vi "Send Set PID Gains Msg.vi"(8 "error in (no error)":errorcluster, 10 "PID gains":T1, 11 "Message Queue in":refnum<queue>) -> (0 "error out":errorcluster, 3 "Message Queue out":refnum<queue>)   [LabVIEW 2024, in "PID Loop.lvlib" / "Set PID Gains Msg.lvclass"]
uses:
  Set PID Gains Msg.lvclass
  Set PID Gains Msg.lvclass/Set PID Gains Msg.ctl
  C:/Users/uspoaotto/OneDrive - Oregon Tool/Desktop/working copies/zeroTimeoutMessageHandler/samples/PID Controller/PID Loop/PID Loop/Set PID Gains Msg/Set PID Gains Msg.lvclass
  C:/Users/uspoaotto/OneDrive - Oregon Tool/Desktop/working copies/zeroTimeoutMessageHandler/src/Zero Timeout Message Handler/~Message/~Message.lvclass
  src/Zero Timeout Message Handler/~Message/~Message.lvclass
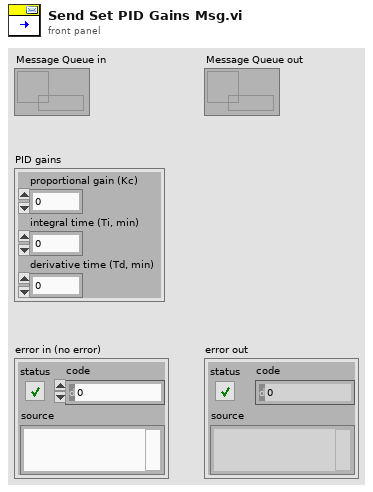
[diagram p1: front panel]
types:
  T1 = cluster{"proportional gain (Kc)":dbl, "integral time (Ti, min)":dbl, "derivative time (Td, min)":dbl}
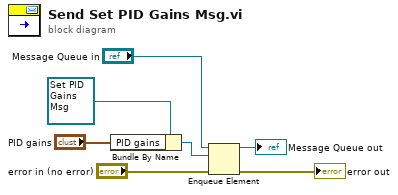
[diagram p0: block diagram]
diagram:
  n1 = Bundle By Name(cluster=refnum<class "Set PID Gains Msg.lvclass"> refnum ("PID Loop.lvlib:Set PID Gains Msg.lvclass"), "PID gains"="PID gains") -> (w1:refnum<class "Set PID Gains Msg.lvclass">)
  n2 = Enqueue Element(queue="Message Queue in", element=w1, error in (no error)="error in (no error)") -> (queue out=→"Message Queue out":refnum<queue>, error out=→"error out":errorcluster)  [unwired: 1 in, 1 out]
